vi "Init.vi"(8 "error in (no error)":errorcluster, 11 "reference in":refnum<class "Barcode_Reader_Dialog.lvclass">) -> (0 "error out":errorcluster, 3 "reference out":refnum<class "Barcode_Reader_Dialog.lvclass">)   [LabVIEW 2022 SP3, in "Barcode_Reader_Dialog.lvlib" / "Barcode_Reader_Dialog.lvclass"]
uses:
  Barcode_Reader_Dialog.lvclass
  Components/Barcode_Reader_Base.lvlibp/Barcode_Reader_Base.lvclass
  Components/ViPER.lvlibp/ViPER.lvclass
  C:/Projects/Medulla/ViPER/Examples/Flux_Capacitor_Tester/Components/ViPER.lvlibp/ViPER.lvclass
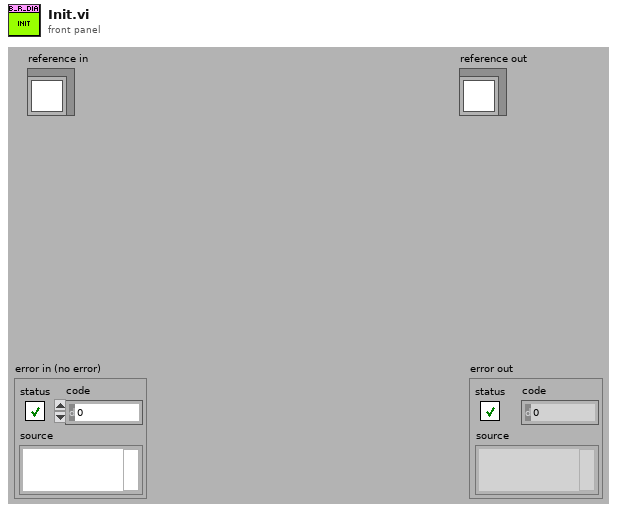
[diagram p1: front panel]
types:
  T1 = typedef "Barcode_Reader_Dialog.lvlib/Barcode_Reader_Dialog.lvclass/ObjectAttributes.ctl" = cluster{"Config":T2, "Serial":string}
  T2 = typedef "Barcode_Reader_Dialog.lvlib/Barcode_Reader_Dialog.lvclass/Config.ctl" = cluster{"default":string}
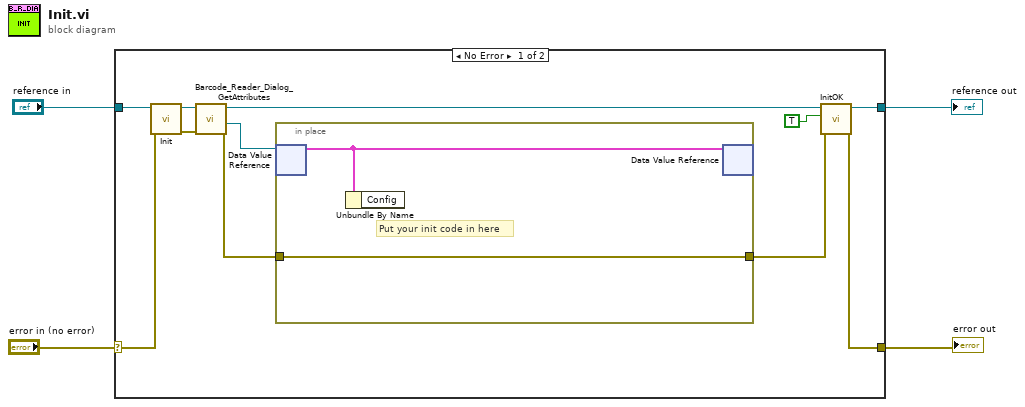
[diagram p0: block diagram]
diagram:
  n1 = case shown="No Error" "error in (no error)" {
    selector: "error in (no error)" -> [w14 w19]
    tunnel: [w5 w19] -> w3
    tunnel: [w8 w18] -> w1
    tunnel: "reference in" -> [w15 w18]
    frame No Error {
      n2 = call-parent "Init.vi"("error in (no error)"=w14, "reference in"=w15) -> ("error out"=w12:errorcluster, "reference out"=w13:refnum<class "Barcode_Reader_Dialog.lvclass">)  [unwired: 8 in]
      n3 = call "Barcode_Reader_Dialog_GetAttributes.vi"("error in (no error)"=w12, "reference in"=w13) -> ("error out"=w10:errorcluster, "DataRef"=w11:refnum<data-value>, "reference out"=w9:refnum<class "Barcode_Reader_Dialog.lvclass">)  [unwired: 6 in, 1 out]
      n4 = in-place {
        in-place-border: w10 -> [w17]
        in-place-border: [w17] -> w6
        # "Put your init code in here"
        n5 = in-place-dvr #1(w11) -> (w16:T1)  [unwired: 1 out]
        n6 = Unbundle By Name(w16) -> ()  [unwired: 1 out]
        n7 = in-place-dvr #1(w16) -> ()  [unwired: 2 out]
      }
      n8 = call "InitOK.vi"("error in (no error)"=w6, "Init OK?"=TRUE, "reference in"=w9) -> ("error out"=w5:errorcluster, "reference out"=w8:refnum<class "Barcode_Reader_Dialog.lvclass">)  [unwired: 7 in]
    }
    frame Error {
    }
  }
  "error out" <- w3
  "reference out" <- w1
